vi "Read Settings Button.vi"(8 "error in (no error)":errorcluster, 11 "UI in":refnum<class "UI.lvclass">) -> (0 "error out":errorcluster, 2 "Settings Button":refnum<vi>, 3 "UI out":refnum<class "UI.lvclass">)   [LabVIEW 2017, in "Generic UI Actor.lvlib" / "UI.lvclass"]
uses:
  UI.lvclass
  UI.lvclass/UI.ctl
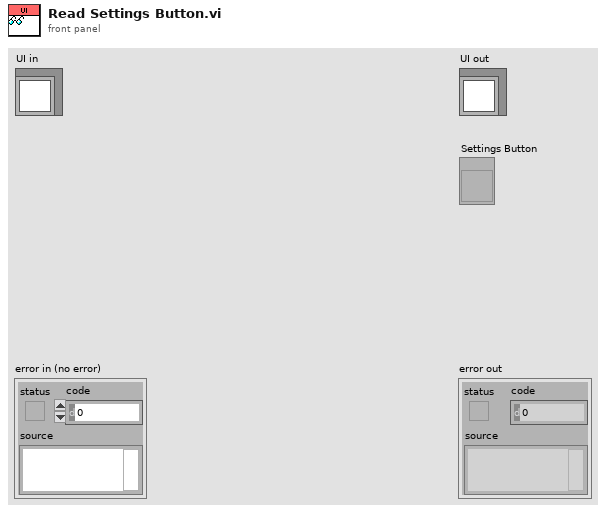
[diagram p1: front panel]
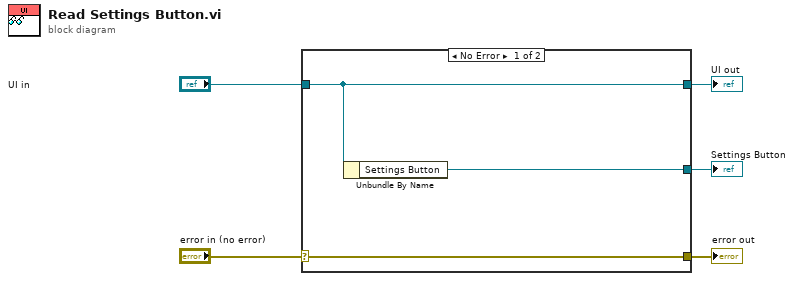
[diagram p0: block diagram]
diagram:
  n1 = case shown="No Error" "error in (no error)" {
    selector: "error in (no error)" -> [w8 w9]
    tunnel: [w8 w9] -> w4
    tunnel: [w7 w10] -> w2
    tunnel: "UI in" -> [w7 w10]
    tunnel: [w6 _] -> w1
    frame No Error {
      n2 = Unbundle By Name(w7) -> ("Settings Button"=w6:refnum<vi>)
    }
    frame Error {
    }
  }
  "error out" <- w4
  "UI out" <- w2
  "Settings Button" <- w1
